vi "Temperature Calculations.vi"(6 "Conversion":dbl, 7 "Slide Refnum":refnum<vi>, 8 "error in":errorcluster, 9 "Image Pixels (U16)":u16[][](array[numeric]), 10 "Last Mouse Position:All Elements In":cluster{"X":i32, "Y":i32}, 11 "Image In":T1) -> (0 "error out":errorcluster, 1 "Temp Array":dbl[][](array[numeric]), 2 "Last Mouse Position:All Elements Out":cluster{"X":i32, "Y":i32}, 3 "Image Out":T1, 4 "Temperature":dbl(slide) scale=21.5..33.60000000000002)   [LabVIEW 2023]
doc: "Calculates the temperature into Celsius from mouse position within the Image Indicator."
uses:
  <vilib>/vision/Image Controls.llb/IMAQ Image.ctl
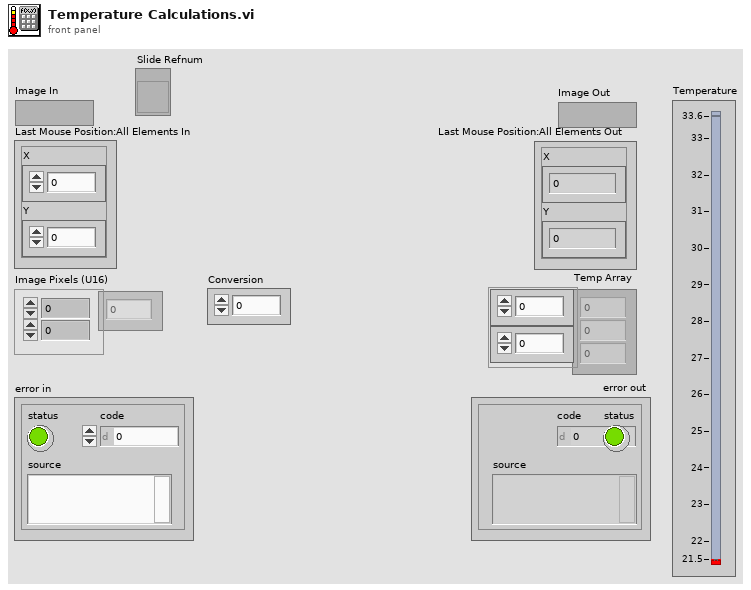
[diagram p1: front panel]
types:
  T1 = typedef "IMAQ Image.ctl" = refnum<image>
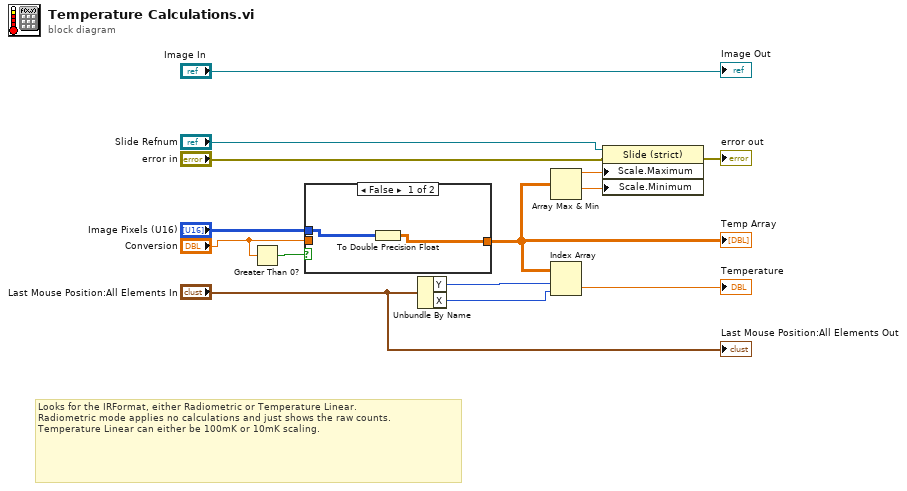
[diagram p0: block diagram]
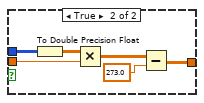
[diagram p2: hidden frame]
diagram:
  # "Looks for the IRFormat, either Radiometric or Temperature Linear. \nRadiometric mode applies no calculations and just shows the raw counts.\nTemperature Linear can either be 100mK or 10mK scaling."
  n1 = Greater Than 0?(x="Conversion") -> (x > 0?=w1:bool)
  n2 = case shown="False" w1 {
    tunnel: "Image Pixels (U16)" -> [w16 w19]
    tunnel: [w15 w18] -> w10
    tunnel: "Conversion" -> [_ w17]
    frame False {
      n3 = To Double Precision Float(number=w16) -> (double precision float=w15:dbl[][])
    }
    frame True {
      n4 = To Double Precision Float(number=w19) -> (double precision float=w22:dbl[][])
      n5 = Multiply(x=w22, y=w17) -> (x*y=w20:dbl[][])
      n6 = Subtract(x=w20, y=273.0) -> (x-y=w18:dbl[][])
    }
  }
  "Temp Array" <- w10
  n7 = Unbundle By Name("Last Mouse Position:All Elements In") -> ("Y"=w12:i32, "X"=w13:i32)
  n8 = Array Max & Min(array=w10) -> (max value=w7:dbl, min value=w6:dbl)  [unwired: 2 out]
  n9 = Index Array(array=w10, index (row)=w12, index (col)=w13) -> (element=→"Temperature":dbl)
  n10 = property class="Slide (strict)"(reference="Slide Refnum", error in="error in", "Scale.Maximum"=w7, "Scale.Minimum"=w6) -> (error out=→"error out":errorcluster)  [unwired: 1 out]
  "Last Mouse Position:All Elements Out" <- "Last Mouse Position:All Elements In"
  "Image Out" <- "Image In"
